vi "Hausmodell.Raumtemperatur.vi"(8 "Error IN":errorcluster, 9 "Solare Gewinne [W/m2]":dbl, 10 "Aussentemperatur [°C]":dbl, 11 "Hausmodell IN":refnum<data-value>) -> (0 "Error OUT":errorcluster, 3 "Hausmodell OUT":refnum<data-value>)   [LabVIEW 2016, in "Hausmodell.lvclass"]
uses:
  Hausmodell.lvclass
  Hausmodell.lvclass/Hausmodell.ctl
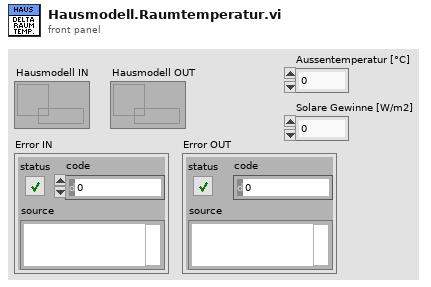
[diagram p1: front panel]
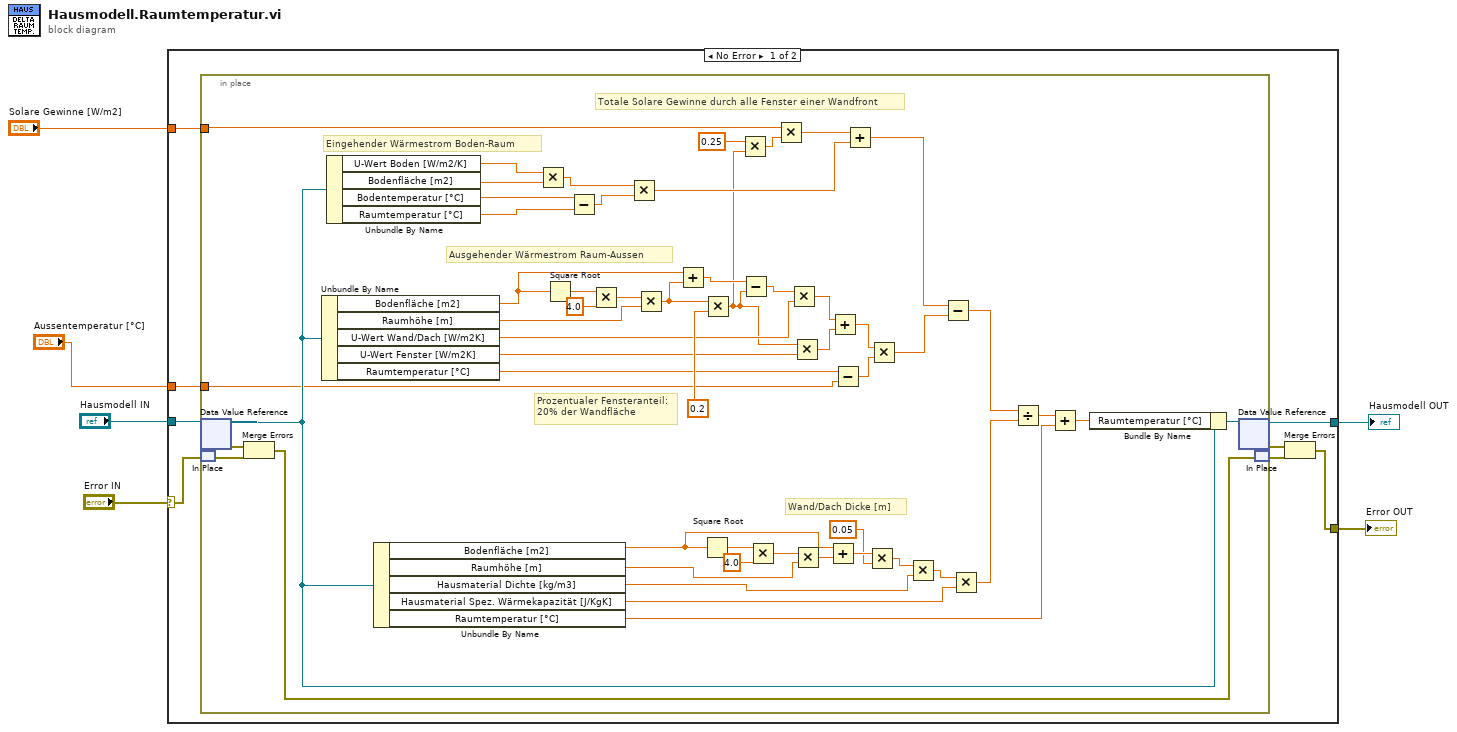
[diagram p0: block diagram]
diagram:
  n1 = case shown="No Error" "Error IN" {
    selector: "Error IN" -> [w12 w69]
    tunnel: [w14 w68] -> w6
    tunnel: "Hausmodell IN" -> [w13 w68]
    tunnel: [w10 w69] -> w4
    tunnel: "Aussentemperatur [°C]" -> [w8 _]
    tunnel: "Solare Gewinne [W/m2]" -> [w7 _]
    frame No Error {
      n2 = in-place {
        in-place-border: w8 -> [w22]
        in-place-border: w7 -> [w19]
        # "Totale Solare Gewinne durch alle Fenster einer Wandfront"
        # "Ausgehender Wärmestrom Raum-Aussen"
        # "Prozentualer Fensteranteil:\n20% der Wandfläche"
        # "Eingehender Wärmestrom Boden-Raum"
        # "Wand/Dach Dicke [m]"
        n3 = in-place-dvr #1(w13) -> (w56:refnum<class "Hausmodell.lvclass">, w66:errorcluster)
        n4 = in-place-match #2(w12) -> (w65:errorcluster)
        n5 = Merge Errors(w66, w65) -> (w64:errorcluster)
        n6 = Unbundle By Name(w56) -> ("Bodenfläche [m2]"=w32:dbl, "Raumhöhe [m]"=w35:dbl, "U-Wert Wand/Dach [W/m2K]"=w29:dbl, "U-Wert Fenster [W/m2K]"=w28:dbl, "Raumtemperatur [°C]"=w23:dbl)
        n7 = Unbundle By Name(w56) -> ("U-Wert Boden [W/m2/K]"=w63:dbl, "Bodenfläche [m2]"=w62:dbl, "Bodentemperatur [°C]"=w61:dbl, "Raumtemperatur [°C]"=w60:dbl)
        n8 = Unbundle By Name(w56) -> ("Bodenfläche [m2]"=w50:dbl, "Raumhöhe [m]"=w52:dbl, "Hausmaterial Dichte [kg/m3]"=w46:dbl, "Hausmaterial Spez. Wärmekapazität [J/KgK]"=w44:dbl, "Raumtemperatur [°C]"=w40:dbl)
        n9 = Multiply(x=w63, y=w62) -> (x*y=w59:dbl)
        n10 = Square Root(x=w32) -> (sqrt(x)=w37:dbl)
        n11 = Subtract(x=w61, y=w60) -> (x-y=w58:dbl)
        n12 = Multiply(x=w37, y=4.0) -> (x*y=w36:dbl)
        n13 = Multiply(x=w59, y=w58) -> (x*y=w21:dbl)
        n14 = Multiply(x=w36, y=w35) -> (x*y=w33:dbl)
        n15 = Add(x=w32, y=w33) -> (x+y=w31:dbl)
        n16 = Square Root(x=w50) -> (sqrt(x)=w54:dbl)
        n17 = Multiply(x=w33, y=0.2) -> (x*y=w18:dbl)
        n18 = Multiply(x=0.25, y=w18) -> (x*y=w17:dbl)
        n19 = Subtract(x=w31, y=w18) -> (x-y=w30:dbl)
        n20 = Multiply(x=w54, y=4.0) -> (x*y=w53:dbl)
        n21 = Multiply(x=w19, y=w17) -> (x*y=w15:dbl)
        n22 = Multiply(x=w30, y=w29) -> (x*y=w27:dbl)
        n23 = Multiply(x=w18, y=w28) -> (x*y=w26:dbl)
        n24 = Multiply(x=w53, y=w52) -> (x*y=w51:dbl)
        n25 = Add(x=w50, y=w51) -> (x+y=w49:dbl)
        n26 = Add(x=w27, y=w26) -> (x+y=w25:dbl)
        n27 = Subtract(x=w23, y=w22) -> (x-y=w24:dbl)
        n28 = Add(x=w15, y=w21) -> (x+y=w20:dbl)
        n29 = Multiply(x=w49, y=0.05) -> (x*y=w47:dbl)
        n30 = Multiply(x=w25, y=w24) -> (x*y=w57:dbl)
        n31 = Multiply(x=w47, y=w46) -> (x*y=w45:dbl)
        n32 = Subtract(x=w20, y=w57) -> (x-y=w43:dbl)
        n33 = Multiply(x=w45, y=w44) -> (x*y=w42:dbl)
        n34 = Divide(x=w43, y=w42) -> (x/y=w41:dbl)
        n35 = Add(x=w41, y=w40) -> (x+y=w39:dbl)
        n36 = Bundle By Name(cluster=w56, "Raumtemperatur [°C]"=w39) -> (w67:refnum<class "Hausmodell.lvclass">)
        n37 = in-place-dvr #1(w67) -> (w14:refnum<data-value>, w11:errorcluster)
        n38 = in-place-match #2(w64) -> (w9:errorcluster)
      }
      n39 = Merge Errors(w11, w9) -> (w10:errorcluster)
    }
    frame Error {
    }
  }
  "Hausmodell OUT" <- w6
  "Error OUT" <- w4
